vi "Display Actor Name.vi"(8 "error in":errorcluster, 10 "Appended Message":string, 11 "_Parent Actor Template in":refnum<class "_Parent Actor Template.lvclass">) -> (0 "error out":errorcluster, 3 "_Parent Actor Template out":refnum<class "_Parent Actor Template.lvclass">)   [LabVIEW 2016, in "_Parent Actor Template.lvlib" / "_Parent Actor Template.lvclass"]
doc: "Displays the name of the Actor in a dialog popup."
uses:
  _Parent Actor Template.lvclass
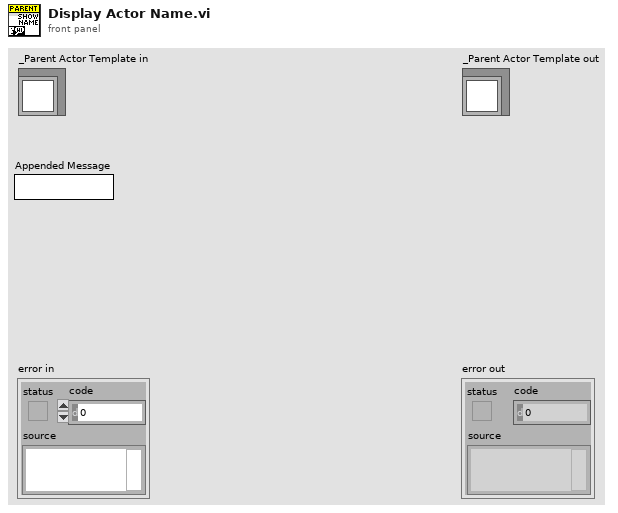
[diagram p1: front panel]
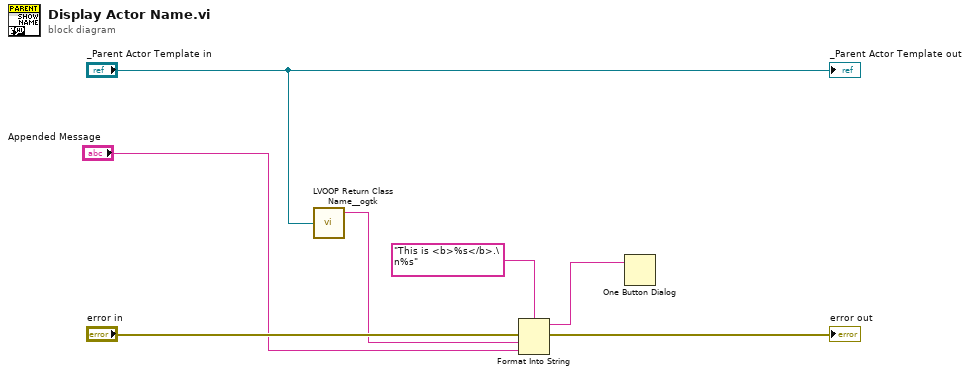
[diagram p0: block diagram]
diagram:
  n1 = call <userlib>:"LVOOP Return Class Name__ogtk.vi"("Object"="_Parent Actor Template in") -> ("Class Base Name"=w5:string)  [unwired: 2 out]
  n2 = Format Into String(format string="This is <b>%s</b>.\n%s", error in="error in", w5, "Appended Message") -> (resulting string=w1:string, error out=→"error out":errorcluster)  [unwired: 1 in]
  n3 = One Button Dialog(message=w1) -> ()  [unwired: 1 in, 1 out]
  "_Parent Actor Template out" <- "_Parent Actor Template in"
